vi "Test Microm sm.vi"() -> ()   [LabVIEW 2024]
uses:
  Micron Optics sm130/Micron Optics sm130.lvlib
panel:
  in  "VISA resource name":refnum<visa-resource-name>
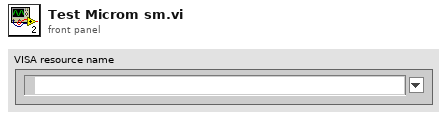
[diagram p1: front panel]
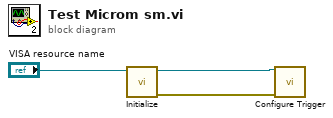
[diagram p0: block diagram]
diagram:
  n1 = call "Initialize.vi"("VISA resource name"="VISA resource name") -> ("error out"=w1:errorcluster, "VISA resource name out"=w2:refnum<visa-resource-name>)  [unwired: 9 in]
  n2 = call "Configure Trigger.vi"("VISA resource name"=w2, "error in (no error)"=w1) -> ()  [unwired: 11 in, 3 out]
